vi "getTypeDescriptor.vi"(8 "error in (no error)":errorcluster, 11 "HGF_SVCommand.lvclass in":refnum<class "HGF_SVCommand.lvclass">) -> (0 "error out":errorcluster, 2 "typeDescriptor":string, 3 "HGF_SVCommand.lvclass out":refnum<class "HGF_SVCommand.lvclass">)   [LabVIEW 2012, in "HGF_SV.lvlib" / "HGF_SVCommand.lvclass"]
uses:
  HGF_SVCommand.lvclass
  HGF_SVCommand.lvclass/HGF_SVCommand.ctl
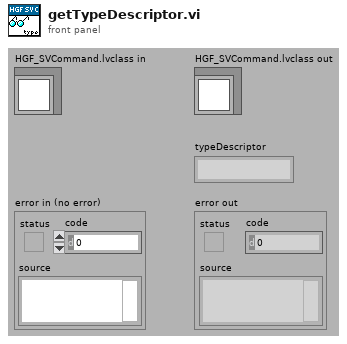
[diagram p1: front panel]
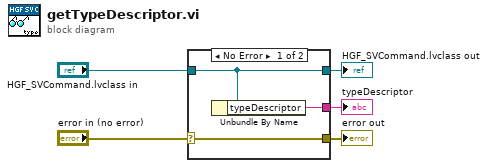
[diagram p0: block diagram]
diagram:
  n1 = case shown="No Error" "error in (no error)" {
    selector: "error in (no error)" -> [w8 w9]
    tunnel: [w8 w9] -> w4
    tunnel: [w7 w10] -> w2
    tunnel: "HGF_SVCommand.lvclass in" -> [w7 w10]
    tunnel: [w6 _] -> w1
    frame No Error {
      n2 = Unbundle By Name(w7) -> ("typeDescriptor"=w6:string)
    }
    frame Error {
    }
  }
  "error out" <- w4
  "HGF_SVCommand.lvclass out" <- w2
  "typeDescriptor" <- w1
